vi "SetValue.vi"(8 "error in":errorcluster, 10 "Value":i64, 11 "Integer in":refnum<class "Integer.lvclass">) -> (0 "error out":errorcluster, 3 "Integer out":refnum<class "Integer.lvclass">)   [LabVIEW 2021, in "ProligentXMLGenerator.lvlib" / "Integer.lvclass"]
uses:
  Integer.lvclass
  Integer.lvclass/Integer.ctl
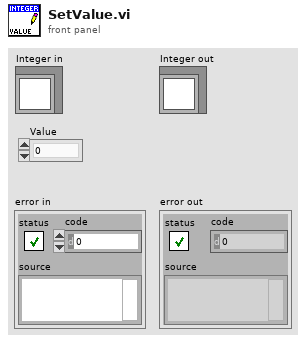
[diagram p1: front panel]
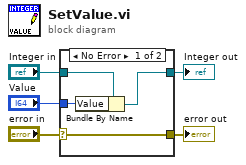
[diagram p0: block diagram]
diagram:
  n1 = case shown="No Error" "error in" {
    selector: "error in" -> [w6 w10]
    tunnel: "Integer in" -> [w9 w11]
    tunnel: [w8 w11] -> w1
    tunnel: "Value" -> [w7 _]
    tunnel: [w6 w10] -> w2
    frame No Error {
      n2 = Bundle By Name(cluster=w9, "Value"=w7) -> (w8:refnum<class "Integer.lvclass">)
    }
    frame Error {
    }
  }
  "error out" <- w2
  "Integer out" <- w1
